vi "util.unit-dose.path-builder.vi"(9 "Unit Index":i32, 10 "Input":string, 11 "Proc Name":string) -> (3 "\\NUTRITION\\ORP\\ORP_U1_2024-08-16.*":string)   [LabVIEW 2024]
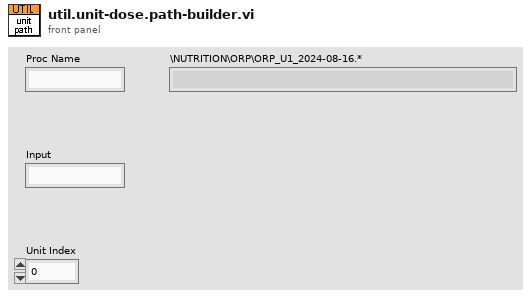
[diagram p1: front panel]
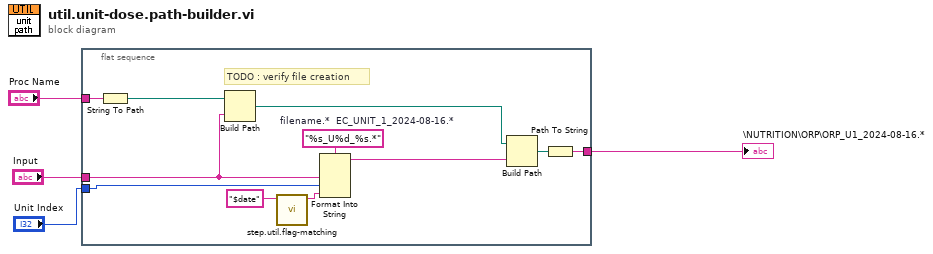
[diagram p0: block diagram]
diagram:
  n1 = flat-sequence {
    tunnel: [w13] -> w4
    tunnel: "Proc Name" -> [w7]
    tunnel: "Unit Index" -> [w6]
    tunnel: "Input" -> [w5]
    frame #0 {
      w14 = "%s_U%d_%s.*"  # filename.*  EC_UNIT_1_2024-08-16.*
      # "TODO : verify file creation"
      n2 = String To Path(string=w7) -> (path=w15:path)
      n3 = Build Path(base path=w15, name or relative path=w5) -> (appended path=w11:path)
      n4 = call "step.util.flag-matching.vi"("$string in"="$date") -> ("formated string out"=w8:string)  [unwired: 10 in]
      n5 = Format Into String(format string=w14, w5, w6, w8) -> (resulting string=w12:string)  [unwired: 2 in, 1 out]
      n6 = Build Path(base path=w11, name or relative path=w12) -> (appended path=w10:path)
      n7 = Path To String(path=w10) -> (string=w13:string)
    }
  }
  "\\NUTRITION\\ORP\\ORP_U1_2024-08-16.*" <- w4
